vi "FastStream.vi"() -> ()   [LabVIEW 2015]
panel:
  out "read buffer":string
  out "Numeric 2":i32
  out "value":i16[](array[numeric]) format="%b"
  in  "Numeric":i32
  in  "VISA Resource Name":refnum<visa-resource-name>
  out "error out":errorcluster
  in  "error in (no error)":errorcluster
  out "appended array 2":dbl[][](array[numeric])
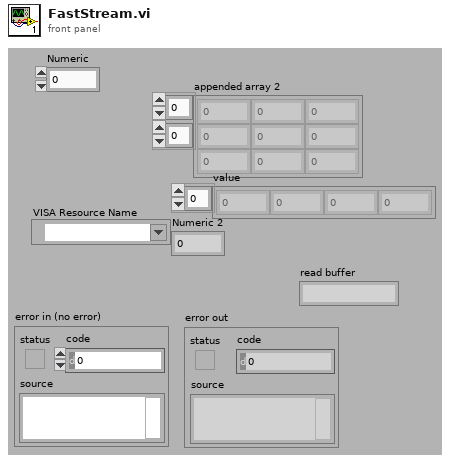
[diagram p1: front panel]
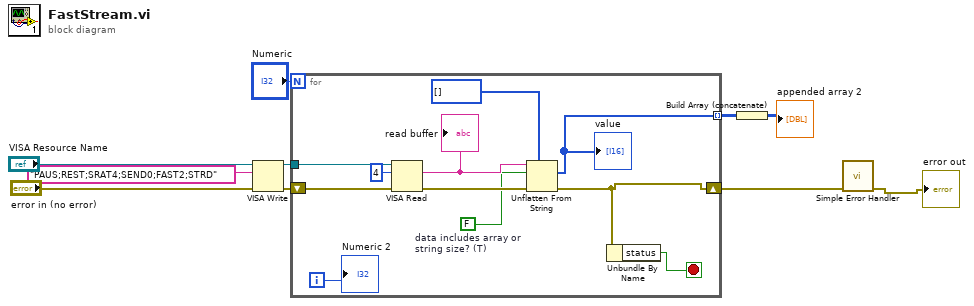
[diagram p0: block diagram]
diagram:
  n1 = VISA Write(VISA resource name="VISA Resource Name", write buffer="PAUS;REST;SRAT4;SEND0;FAST2;STRD", error in (no error)="error in (no error)") -> (VISA resource name out=w8:refnum<visa-resource-name>, error out=w7:errorcluster)  [unwired: 1 out]
  n2 = for {
    N: "Numeric" -> [_]
    shift-right: [w13] -> w3
    shift-left: w7 -> [w21]
    tunnel: w8 -> [w20]
    tunnel: [w14] -> w6 mode=indexing
    i -> [w11]
    stop <- w12 stop-if-true
    w15 = FALSE  # data includes array or string size? (T)
    n3 = VISA Read(VISA resource name=w20, byte count=u32 4, error in (no error)=w21) -> (read buffer=w17:string, error out=w18:errorcluster)  [unwired: 2 out]
    "read buffer" <- w17
    n4 = Unflatten From String(type=i16[] [], binary string=w17, data includes array or string size? (T)=w15, error in (no error)=w18) -> (value=w14:i16[], error out=w13:errorcluster)  [unwired: 2 out]
    "value" <- w14
    n5 = Unbundle By Name(w13) -> ("status"=w12:bool)
    "Numeric 2" <- w11
  }
  n6 = Build Array (concatenate)(w6) -> (→"appended array 2":i16[][])
  n7 = call <vilib>:"Simple Error Handler.vi"("error in (no error)"=w3) -> ("error out"=→"error out":errorcluster)  [unwired: 1 in, 7 out]
